vi "TIO RPC Blocking.vi"(8 "error in (no error)":errorcluster, 9 "Payload":string, 10 "Named Method":string="mcu.desc", 11 "TC Connection":T1={"Type"=enum."Serial", "URL"="serial:///dev/cu.usbserial-00000", "TO"=500, "Addr"=0, "Port"=0, "TCP"=refnum, "UDP"=refnum, "Route"=""}) -> (0 "error out":errorcluster={"status"=TRUE, "code"=-1073807252, "source"="VISA Read in SLIP Decode Serial Read.vi->NN VISA Read.vi->NN RPC.vi"}, 1 "Response":bool, 2 "Respose":string, 3 "TC Connection":T1={"Type"=enum."Serial", "URL"="serial:///dev/cu.usbserial-00000", "TO"=500, "Addr"=0, "Port"=0, "TCP"=refnum, "UDP"=refnum, "Route"=""})   [LabVIEW 2010]
uses:
  <userlib>/TIO Library 2010/TIO RPC Form Request.vi
  <userlib>/TIO Library 2010/TIO Parse Packet.vi
  <userlib>/TIO Library 2010/TIO SLIP Serial Read.vi
  <userlib>/TIO Library 2010/TIO Serial Checksum CRC32.vi
  <userlib>/TIO Library 2010/TIO Stream Write.vi
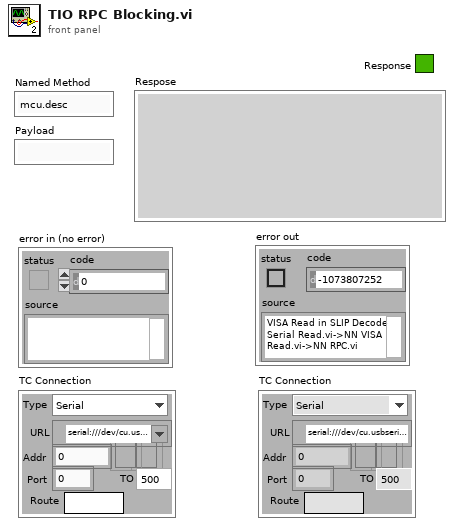
[diagram p1: front panel]
types:
  T1 = cluster{"Type":enum16{"Serial", "TCP", "UDP", "mUDP"}, "URL":refnum<visa-resource-name>, "TO":u32, "Addr":u32, "Port":i32, "TCP":refnum<k5>, "UDP":refnum<k16>, "Route":string}
  T2 = enum8{"Invalid", "Log", "RPC Request", "RPC Reply", "RPC Error", "Stream Description", "User"}
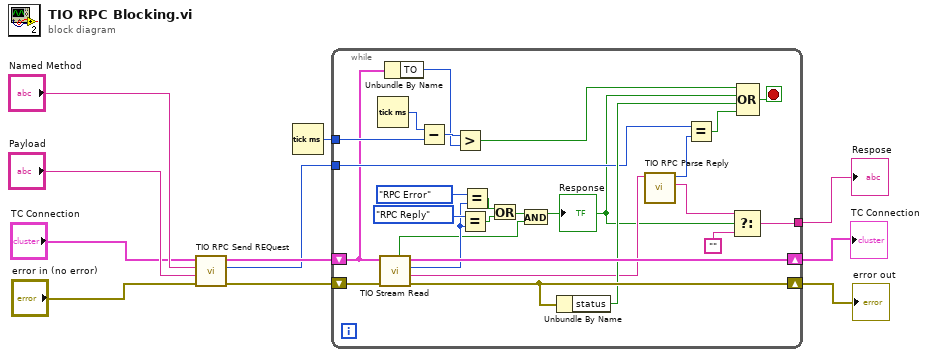
[diagram p0: block diagram]
diagram:
  n1 = call <userlib>:"TIO RPC Send REQuest.vi"("error in (no error)"="error in (no error)", "Payload"="Payload", "Topic"="Named Method", "TC Connection"="TC Connection") -> ("error out"=w11:errorcluster, "Request ID"=w1:u16, "TC Connection"=w9:T1)  [unwired: 5 in]
  n2 = Tick Count (ms)() -> (millisecond timer value=w6:u32)
  n3 = while {
    shift-right: [w32] -> w10
    shift-left: w11 -> [w37]
    shift-right: [w36] -> w3
    shift-left: w9 -> [w15]
    tunnel: w6 -> [w34]
    tunnel: [w26] -> w2
    tunnel: w1 -> [w24]
    stop <- w29 stop-if-true
    n4 = Tick Count (ms)() -> (millisecond timer value=w35:u32)
    n5 = call <userlib>:"TIO Stream Read.vi"("error in (no error)"=w37, "TC Connection"=w15) -> ("error out"=w32:errorcluster, "Payload"=w22:string, "Type"=w18:T2, "TC Connection"=w36:T1, "Routing Matches"=w12:bool)  [unwired: 4 in, 1 out]
    n6 = Unbundle By Name(w15) -> ("TO"=w28:u32)
    n7 = Subtract(x=w35, y=w34) -> (x-y=w33:u32)
    n8 = Greater?(x=w33, y=w28) -> (0:w31:bool)
    n9 = Equal?(x=T2."RPC Reply" ("Type"), y=w18) -> (x = y?=w16:bool)
    n10 = Equal?(x=T2."RPC Error" ("Type"), y=w18) -> (x = y?=w17:bool)
    n11 = Or(x=w17, y=w16) -> (x .or. y?=w14:bool)
    n12 = And(x=w14, y=w12) -> (x .and. y?=w13:bool)
    "Response" <- w13
    n13 = Unbundle By Name(w32) -> ("status"=w30:bool)
    n14 = call <userlib>:"TIO RPC Parse Reply.vi"("Payload"=w22) -> ("Payload"=w20:string, "Request ID"=w21:u16)  [unwired: 9 in]
    n15 = Equal?(x=w24, y=w21) -> (x = y?=w23:bool)
    n16 = Select(t=w20, s=w13, f="") -> (s? t:f=w26:string)
    n17 = Compound Arithmetic op=OR(w31, w13, w30, w23) -> (w29:bool)
  }
  "error out" <- w10
  "Respose" <- w2
  "TC Connection" <- w3
